vi "Update.vi"(8 "error in (no error)":errorcluster, 10 "Time Waited":dbl, 11 "StopInstruction in":refnum<class "StopInstruction.lvclass">) -> (0 "error out":errorcluster, 3 "StopInstruction out":refnum<class "StopInstruction.lvclass">)   [LabVIEW 2015, in "StopInstruction.lvclass"]
uses:
  StopInstruction.lvclass
  StopInstruction.lvclass/StopInstruction.ctl
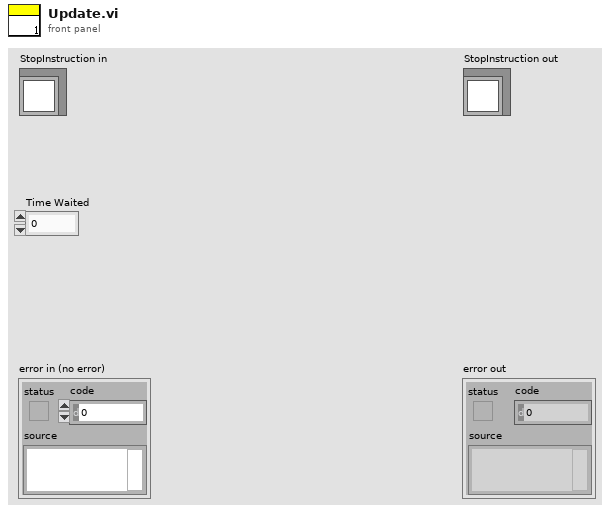
[diagram p1: front panel]
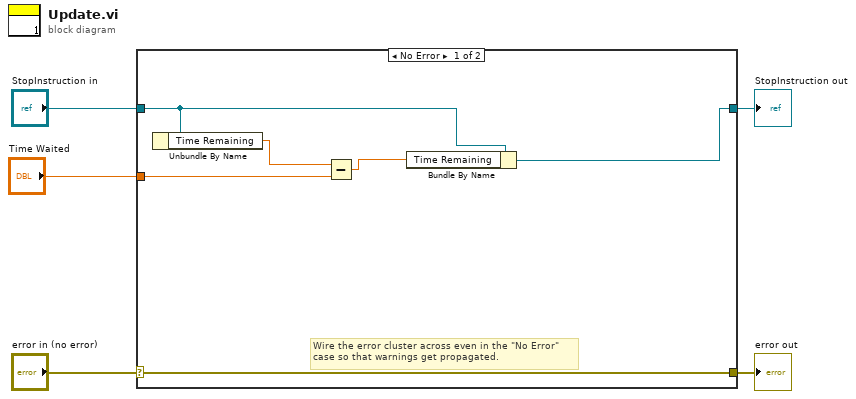
[diagram p0: block diagram]
diagram:
  n1 = case shown="No Error" "error in (no error)" {
    selector: "error in (no error)" -> [w11 w13]
    tunnel: [w11 w13] -> w4
    tunnel: [w6 w12] -> w2
    tunnel: "StopInstruction in" -> [w7 w12]
    tunnel: "Time Waited" -> [w9 _]
    frame No Error {
      # "Wire the error cluster across even in the \"No Error\"\ncase so that warnings get propagated."
      n2 = Unbundle By Name(w7) -> ("Time Remaining"=w10:dbl)
      n3 = Subtract(x=w10, y=w9) -> (x-y=w8:dbl)
      n4 = Bundle By Name(cluster=w7, "Time Remaining"=w8) -> (w6:refnum<class "StopInstruction.lvclass">)
    }
    frame Error {
    }
  }
  "error out" <- w4
  "StopInstruction out" <- w2
